vi "ELVIS III v1.0 Configure PWM.vi"(8 "error in (no error)":errorcluster, 9 "PWM Configuration":T4, 10 "PWM Channel":T1, 11 "myRIO Ref In":T2) -> (0 "error out":errorcluster, 2 "Max Counter Value":u16, 3 "Actual Frequency (Hz)":dbl)   [LabVIEW 2021]
uses:
  <vilib>/myRIO/Common/Instrument Driver Framework/myRIO v1.0/PWM/typedefs/PWM Configuration v1.0.ctl
  <vilib>/myRIO/Common/Instrument Driver Framework/Utilities/typedefs/myRIO v1.0 Reference.ctl
  <vilib>/myRIO/Common/Instrument Driver Framework/Utilities/typedefs/Generic FPGA Reference.ctl
  <vilib>/myRIO/Common/Instrument Driver Framework/myRIO v1.0/PWM/typedefs/PWM Channels Enum.ctl
  <vilib>/myRIO/Common/Instrument Driver Framework/ELVIS III v1.0/PWM/typedefs/ELVIS III PWM Channels FPGA Reference.ctl
  <vilib>/myRIO/Common/Instrument Driver Framework/Utilities/vis/Calculate Clock Settings.vi
  <vilib>/myRIO/Common/Instrument Driver Framework/Utilities/vis/Calculate TOP (Phase Correct Mode).vi
  <vilib>/myRIO/Common/Instrument Driver Framework/Utilities/vis/Calculate TOP (Normal Mode).vi
  <vilib>/myRIO/Common/Instrument Driver Framework/Utilities/vis/Calculate Frequency (Phase Correct Mode).vi
  <vilib>/myRIO/Common/Instrument Driver Framework/Utilities/vis/Calculate Frequency (Normal Mode).vi
  <vilib>/rvi/errors/niLvFpgaAdjustHostInterfaceError.vi
  <vilib>/rvi/interface/nirviReadWriteControl/nirviReadWriteControl.xnode
  NiFpgaLv.dll
  <vilib>/rvi/interface/Simulation/niFpgaSimulationCallBeginRW.vi
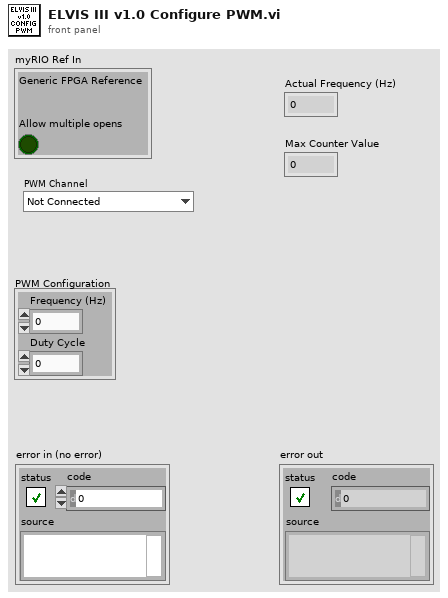
[diagram p1: front panel]
types:
  T1 = typedef "PWM Channels Enum.ctl" = enum16{"Not Connected", "C/PWM0", "C/PWM1", "A/PWM0", "A/PWM1", "A/PWM2", "A/PWM3", "A/PWM4", "A/PWM5", "A/PWM6", "A/PWM7", "A/PWM8", "A/PWM9", "A/PWM10", "A/PWM11", "A/PWM12", "A/PWM13", "A/PWM14", "A/PWM15", "A/PWM16", "A/PWM17", "A/PWM18", "A/PWM19", "B/PWM0", "B/PWM1", "B/PWM2", "B/PWM3", "B/PWM4", "B/PWM5", "B/PWM6", "B/PWM7", "B/PWM8", "B/PWM9", "B/PWM10", "B/PWM11", "B/PWM12", "B/PWM13", "B/PWM14", "B/PWM15", "B/PWM16", "B/PWM17", "B/PWM18", "B/PWM19", "PWM/PWM0", "PWM/PWM1", "PWM/PWM2", "PWM/PWM3", "PWM/PWM4", "PWM/PWM5", "PWM/PWM6", "PWM/PWM7", "PWM/PWM8", "PWM/PWM9"}
  T2 = typedef "myRIO v1.0 Reference.ctl" = cluster{"Generic FPGA Reference":T3, "Allow multiple opens":bool}
  T3 = typedef "Generic FPGA Reference.ctl" = refnum<k20>
  T4 = typedef "PWM Configuration v1.0.ctl" = cluster{"Frequency (Hz)":dbl, "Duty Cycle":dbl}
  T5 = typedef "ELVIS III PWM Channels FPGA Reference.ctl" = refnum<k20>
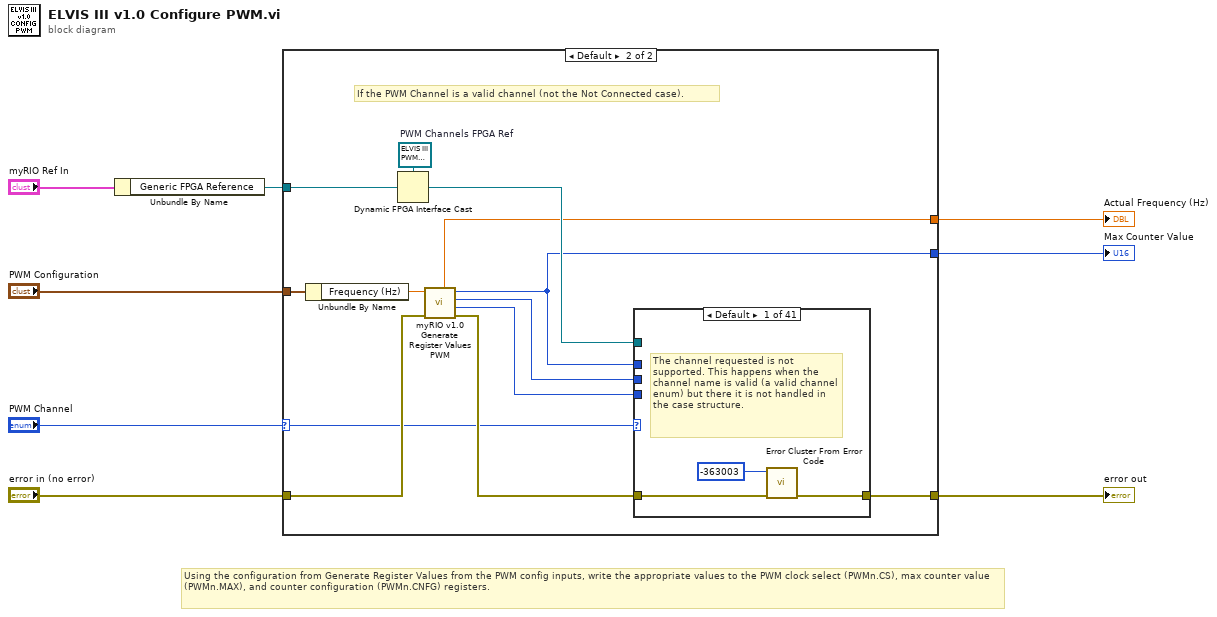
[diagram p0: block diagram]
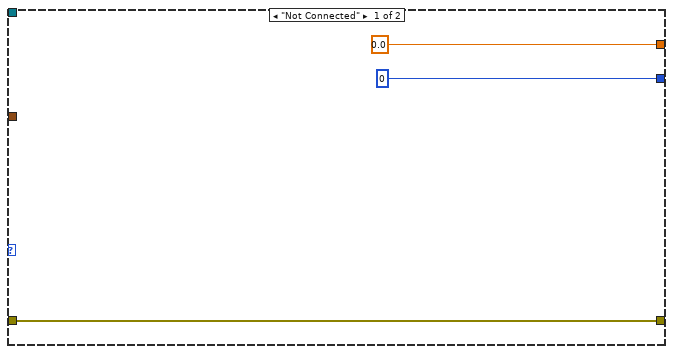
[diagram p2: hidden frame]
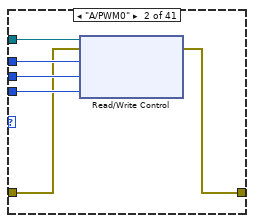
[diagram p3: hidden frame]
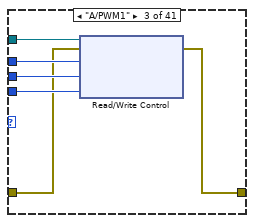
[diagram p4: hidden frame]
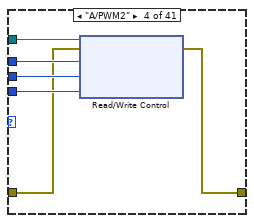
[diagram p5: hidden frame]
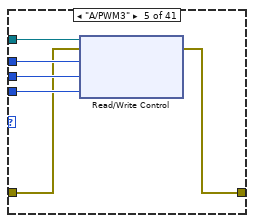
[diagram p6: hidden frame]
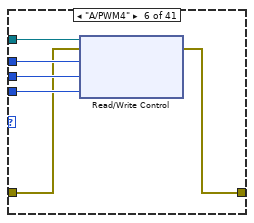
[diagram p7: hidden frame]
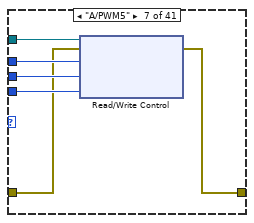
[diagram p8: hidden frame]
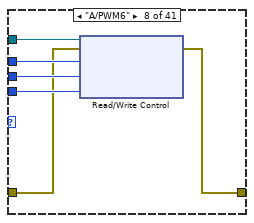
[diagram p9: hidden frame]
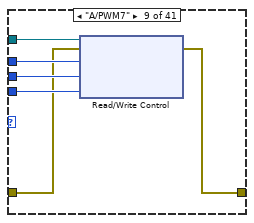
[diagram p10: hidden frame]
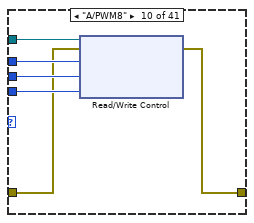
[diagram p11: hidden frame]
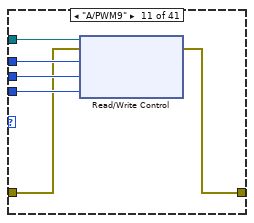
[diagram p12: hidden frame]
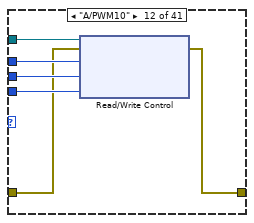
[diagram p13: hidden frame]
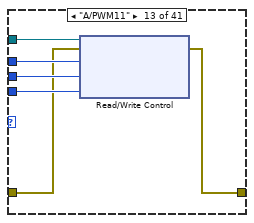
[diagram p14: hidden frame]
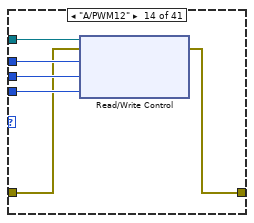
[diagram p15: hidden frame]
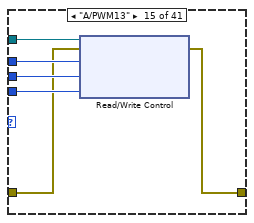
[diagram p16: hidden frame]
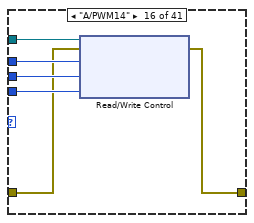
[diagram p17: hidden frame]
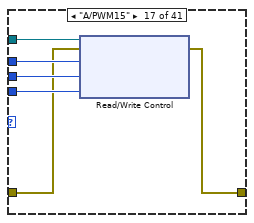
[diagram p18: hidden frame]
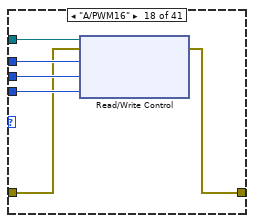
[diagram p19: hidden frame]
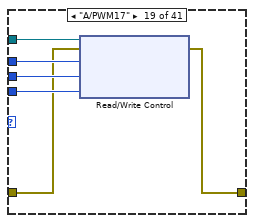
[diagram p20: hidden frame]
diagram:
  # "Using the configuration from Generate Register Values from the PWM config inputs, write the appropriate values to the PWM clock select (PWMn.CS), max counter value (PWMn.MAX), and counter configuration (PWMn.CNFG) registers."
  n1 = Unbundle By Name("myRIO Ref In") -> ("Generic FPGA Reference"=w1:T3)
  n2 = case shown="Default" "PWM Channel" {
    selector: "PWM Channel" -> [_ w12]
    tunnel: [w9 w22] -> w8
    tunnel: "PWM Configuration" -> [_ w14]
    tunnel: "error in (no error)" -> [w9 w16]
    tunnel: w1 -> [_ w21]
    tunnel: [u16 0 w19] -> w2
    tunnel: [0.0 ("Actual Frequency (Hz)") w20] -> w3
    frame "Not Connected" {
    }
    frame Default {
      w24 = T5 refnum  # PWM Channels FPGA Ref
      # "If the PWM Channel is a valid channel (not the Not Connected case)."
      n3 = Unbundle By Name(w14) -> ("Frequency (Hz)"=w13:dbl)
      n4 = Dynamic FPGA Interface Cast(Session In=w24, Type=w21) -> (Session Out=w23:T5)
      n5 = call <vilib>:"myRIO v1.0 Generate Register Values PWM.vi"("error in (no error)"=w16, "Frequency (Hz)"=w13) -> ("error out"=w15:errorcluster, "PWM.CS"=w17:u8, "PWM.CNFG"=w18:u8, "PWM.MAX"=w19:u16, "Actual Frequency (Hz)"=w20:dbl)  [unwired: 5 in]
      n6 = case shown="Default" w12 {
        tunnel: w23 -> [_ w33 w39 w45 w51 w57 w63 w69 w75 w81 w87 w93 w99 w105 w111 w117 w123 w129 w135 w141 w147 w153 w159 w165 w171 w177 w183 w189 w195 w201 w207 w213 w219 w225 w231 w237 w243 w249 w255 w261 w267]
        tunnel: [w25 w32 w38 w44 w50 w56 w62 w68 w74 w80 w86 w92 w98 w104 w110 w116 w122 w128 w134 w140 w146 w152 w158 w164 w170 w176 w182 w188 w194 w200 w206 w212 w218 w224 w230 w236 w242 w248 w254 w260 w266] -> w22
        tunnel: w19 -> [_ w31 w37 w43 w49 w55 w61 w67 w73 w79 w85 w91 w97 w103 w109 w115 w121 w127 w133 w139 w145 w151 w157 w163 w169 w175 w181 w187 w193 w199 w205 w211 w217 w223 w229 w235 w241 w247 w253 w259 w265]
        tunnel: w18 -> [_ w30 w36 w42 w48 w54 w60 w66 w72 w78 w84 w90 w96 w102 w108 w114 w120 w126 w132 w138 w144 w150 w156 w162 w168 w174 w180 w186 w192 w198 w204 w210 w216 w222 w228 w234 w240 w246 w252 w258 w264]
        tunnel: w17 -> [_ w29 w35 w41 w47 w53 w59 w65 w71 w77 w83 w89 w95 w101 w107 w113 w119 w125 w131 w137 w143 w149 w155 w161 w167 w173 w179 w185 w191 w197 w203 w209 w215 w221 w227 w233 w239 w245 w251 w257 w263]
        tunnel: w15 -> [w26 w28 w34 w40 w46 w52 w58 w64 w70 w76 w82 w88 w94 w100 w106 w112 w118 w124 w130 w136 w142 w148 w154 w160 w166 w172 w178 w184 w190 w196 w202 w208 w214 w220 w226 w232 w238 w244 w250 w256 w262]
        frame Default {
          # "The channel requested is not supported. This happens when the channel name is valid (a valid channel enum) but there it is not handled in the case structure."
          n7 = call <vilib>:"Error Cluster From Error Code.vi"("error in (no error)"=w26, "error code (0)"=-363003) -> ("error out"=w25:errorcluster)  [unwired: 7 in]
        }
        frame "A/PWM0" {
          n8 = xnode "Read/Write Control"("FPGA VI Reference In"=w33, "error in"=w28, "PWM.A_0.MAX"=w31, "PWM.A_0.CNFG"=w30, "PWM.A_0.CS"=w29) -> ("error out"=w32:errorcluster)  [unwired: 1 out]
        }
        frame "A/PWM1" {
          n9 = xnode "Read/Write Control"("FPGA VI Reference In"=w39, "error in"=w34, "PWM.A_1.MAX"=w37, "PWM.A_1.CNFG"=w36, "PWM.A_1.CS"=w35) -> ("error out"=w38:errorcluster)  [unwired: 1 out]
        }
        frame "A/PWM2" {
          n10 = xnode "Read/Write Control"("FPGA VI Reference In"=w45, "error in"=w40, "PWM.A_2.MAX"=w43, "PWM.A_2.CNFG"=w42, "PWM.A_2.CS"=w41) -> ("error out"=w44:errorcluster)  [unwired: 1 out]
        }
        frame "A/PWM3" {
          n11 = xnode "Read/Write Control"("FPGA VI Reference In"=w51, "error in"=w46, "PWM.A_3.MAX"=w49, "PWM.A_3.CNFG"=w48, "PWM.A_3.CS"=w47) -> ("error out"=w50:errorcluster)  [unwired: 1 out]
        }
        frame "A/PWM4" {
          n12 = xnode "Read/Write Control"("FPGA VI Reference In"=w57, "error in"=w52, "PWM.A_4.MAX"=w55, "PWM.A_4.CNFG"=w54, "PWM.A_4.CS"=w53) -> ("error out"=w56:errorcluster)  [unwired: 1 out]
        }
        frame "A/PWM5" {
          n13 = xnode "Read/Write Control"("FPGA VI Reference In"=w63, "error in"=w58, "PWM.A_5.MAX"=w61, "PWM.A_5.CNFG"=w60, "PWM.A_5.CS"=w59) -> ("error out"=w62:errorcluster)  [unwired: 1 out]
        }
        frame "A/PWM6" {
          n14 = xnode "Read/Write Control"("FPGA VI Reference In"=w69, "error in"=w64, "PWM.A_6.MAX"=w67, "PWM.A_6.CNFG"=w66, "PWM.A_6.CS"=w65) -> ("error out"=w68:errorcluster)  [unwired: 1 out]
        }
        frame "A/PWM7" {
          n15 = xnode "Read/Write Control"("FPGA VI Reference In"=w75, "error in"=w70, "PWM.A_7.MAX"=w73, "PWM.A_7.CNFG"=w72, "PWM.A_7.CS"=w71) -> ("error out"=w74:errorcluster)  [unwired: 1 out]
        }
        frame "A/PWM8" {
          n16 = xnode "Read/Write Control"("FPGA VI Reference In"=w81, "error in"=w76, "PWM.A_8.MAX"=w79, "PWM.A_8.CNFG"=w78, "PWM.A_8.CS"=w77) -> ("error out"=w80:errorcluster)  [unwired: 1 out]
        }
        frame "A/PWM9" {
          n17 = xnode "Read/Write Control"("FPGA VI Reference In"=w87, "error in"=w82, "PWM.A_9.MAX"=w85, "PWM.A_9.CNFG"=w84, "PWM.A_9.CS"=w83) -> ("error out"=w86:errorcluster)  [unwired: 1 out]
        }
        frame "A/PWM10" {
          n18 = xnode "Read/Write Control"("FPGA VI Reference In"=w93, "error in"=w88, "PWM.A_10.MAX"=w91, "PWM.A_10.CNFG"=w90, "PWM.A_10.CS"=w89) -> ("error out"=w92:errorcluster)  [unwired: 1 out]
        }
        frame "A/PWM11" {
          n19 = xnode "Read/Write Control"("FPGA VI Reference In"=w99, "error in"=w94, "PWM.A_11.MAX"=w97, "PWM.A_11.CNFG"=w96, "PWM.A_11.CS"=w95) -> ("error out"=w98:errorcluster)  [unwired: 1 out]
        }
        frame "A/PWM12" {
          n20 = xnode "Read/Write Control"("FPGA VI Reference In"=w105, "error in"=w100, "PWM.A_12.MAX"=w103, "PWM.A_12.CNFG"=w102, "PWM.A_12.CS"=w101) -> ("error out"=w104:errorcluster)  [unwired: 1 out]
        }
        frame "A/PWM13" {
          n21 = xnode "Read/Write Control"("FPGA VI Reference In"=w111, "error in"=w106, "PWM.A_13.MAX"=w109, "PWM.A_13.CNFG"=w108, "PWM.A_13.CS"=w107) -> ("error out"=w110:errorcluster)  [unwired: 1 out]
        }
        frame "A/PWM14" {
          n22 = xnode "Read/Write Control"("FPGA VI Reference In"=w117, "error in"=w112, "PWM.A_14.MAX"=w115, "PWM.A_14.CNFG"=w114, "PWM.A_14.CS"=w113) -> ("error out"=w116:errorcluster)  [unwired: 1 out]
        }
        frame "A/PWM15" {
          n23 = xnode "Read/Write Control"("FPGA VI Reference In"=w123, "error in"=w118, "PWM.A_15.MAX"=w121, "PWM.A_15.CNFG"=w120, "PWM.A_15.CS"=w119) -> ("error out"=w122:errorcluster)  [unwired: 1 out]
        }
        frame "A/PWM16" {
          n24 = xnode "Read/Write Control"("FPGA VI Reference In"=w129, "error in"=w124, "PWM.A_16.MAX"=w127, "PWM.A_16.CNFG"=w126, "PWM.A_16.CS"=w125) -> ("error out"=w128:errorcluster)  [unwired: 1 out]
        }
        frame "A/PWM17" {
          n25 = xnode "Read/Write Control"("FPGA VI Reference In"=w135, "error in"=w130, "PWM.A_17.MAX"=w133, "PWM.A_17.CNFG"=w132, "PWM.A_17.CS"=w131) -> ("error out"=w134:errorcluster)  [unwired: 1 out]
        }
        frame "A/PWM18" {
          n26 = xnode "Read/Write Control"("FPGA VI Reference In"=w141, "error in"=w136, "PWM.A_18.MAX"=w139, "PWM.A_18.CNFG"=w138, "PWM.A_18.CS"=w137) -> ("error out"=w140:errorcluster)  [unwired: 1 out]
        }
        frame "A/PWM19" {
          n27 = xnode "Read/Write Control"("FPGA VI Reference In"=w147, "error in"=w142, "PWM.A_19.MAX"=w145, "PWM.A_19.CNFG"=w144, "PWM.A_19.CS"=w143) -> ("error out"=w146:errorcluster)  [unwired: 1 out]
        }
        frame "B/PWM0" {
          n28 = xnode "Read/Write Control"("FPGA VI Reference In"=w153, "error in"=w148, "PWM.B_0.MAX"=w151, "PWM.B_0.CNFG"=w150, "PWM.B_0.CS"=w149) -> ("error out"=w152:errorcluster)  [unwired: 1 out]
        }
        frame "B/PWM1" {
          n29 = xnode "Read/Write Control"("FPGA VI Reference In"=w159, "error in"=w154, "PWM.B_1.MAX"=w157, "PWM.B_1.CNFG"=w156, "PWM.B_1.CS"=w155) -> ("error out"=w158:errorcluster)  [unwired: 1 out]
        }
        frame "B/PWM2" {
          n30 = xnode "Read/Write Control"("FPGA VI Reference In"=w165, "error in"=w160, "PWM.B_2.MAX"=w163, "PWM.B_2.CNFG"=w162, "PWM.B_2.CS"=w161) -> ("error out"=w164:errorcluster)  [unwired: 1 out]
        }
        frame "B/PWM3" {
          n31 = xnode "Read/Write Control"("FPGA VI Reference In"=w171, "error in"=w166, "PWM.B_3.MAX"=w169, "PWM.B_3.CNFG"=w168, "PWM.B_3.CS"=w167) -> ("error out"=w170:errorcluster)  [unwired: 1 out]
        }
        frame "B/PWM4" {
          n32 = xnode "Read/Write Control"("FPGA VI Reference In"=w177, "error in"=w172, "PWM.B_4.MAX"=w175, "PWM.B_4.CNFG"=w174, "PWM.B_4.CS"=w173) -> ("error out"=w176:errorcluster)  [unwired: 1 out]
        }
        frame "B/PWM5" {
          n33 = xnode "Read/Write Control"("FPGA VI Reference In"=w183, "error in"=w178, "PWM.B_5.MAX"=w181, "PWM.B_5.CNFG"=w180, "PWM.B_5.CS"=w179) -> ("error out"=w182:errorcluster)  [unwired: 1 out]
        }
        frame "B/PWM6" {
          n34 = xnode "Read/Write Control"("FPGA VI Reference In"=w189, "error in"=w184, "PWM.B_6.MAX"=w187, "PWM.B_6.CNFG"=w186, "PWM.B_6.CS"=w185) -> ("error out"=w188:errorcluster)  [unwired: 1 out]
        }
        frame "B/PWM7" {
          n35 = xnode "Read/Write Control"("FPGA VI Reference In"=w195, "error in"=w190, "PWM.B_7.MAX"=w193, "PWM.B_7.CNFG"=w192, "PWM.B_7.CS"=w191) -> ("error out"=w194:errorcluster)  [unwired: 1 out]
        }
        frame "B/PWM8" {
          n36 = xnode "Read/Write Control"("FPGA VI Reference In"=w201, "error in"=w196, "PWM.B_8.MAX"=w199, "PWM.B_8.CNFG"=w198, "PWM.B_8.CS"=w197) -> ("error out"=w200:errorcluster)  [unwired: 1 out]
        }
        frame "B/PWM9" {
          n37 = xnode "Read/Write Control"("FPGA VI Reference In"=w207, "error in"=w202, "PWM.B_9.MAX"=w205, "PWM.B_9.CNFG"=w204, "PWM.B_9.CS"=w203) -> ("error out"=w206:errorcluster)  [unwired: 1 out]
        }
        frame "B/PWM10" {
          n38 = xnode "Read/Write Control"("FPGA VI Reference In"=w213, "error in"=w208, "PWM.B_10.MAX"=w211, "PWM.B_10.CNFG"=w210, "PWM.B_10.CS"=w209) -> ("error out"=w212:errorcluster)  [unwired: 1 out]
        }
        frame "B/PWM11" {
          n39 = xnode "Read/Write Control"("FPGA VI Reference In"=w219, "error in"=w214, "PWM.B_11.MAX"=w217, "PWM.B_11.CNFG"=w216, "PWM.B_11.CS"=w215) -> ("error out"=w218:errorcluster)  [unwired: 1 out]
        }
        frame "B/PWM12" {
          n40 = xnode "Read/Write Control"("FPGA VI Reference In"=w225, "error in"=w220, "PWM.B_12.MAX"=w223, "PWM.B_12.CNFG"=w222, "PWM.B_12.CS"=w221) -> ("error out"=w224:errorcluster)  [unwired: 1 out]
        }
        frame "B/PWM13" {
          n41 = xnode "Read/Write Control"("FPGA VI Reference In"=w231, "error in"=w226, "PWM.B_13.MAX"=w229, "PWM.B_13.CNFG"=w228, "PWM.B_13.CS"=w227) -> ("error out"=w230:errorcluster)  [unwired: 1 out]
        }
        frame "B/PWM14" {
          n42 = xnode "Read/Write Control"("FPGA VI Reference In"=w237, "error in"=w232, "PWM.B_14.MAX"=w235, "PWM.B_14.CNFG"=w234, "PWM.B_14.CS"=w233) -> ("error out"=w236:errorcluster)  [unwired: 1 out]
        }
        frame "B/PWM15" {
          n43 = xnode "Read/Write Control"("FPGA VI Reference In"=w243, "error in"=w238, "PWM.B_15.MAX"=w241, "PWM.B_15.CNFG"=w240, "PWM.B_15.CS"=w239) -> ("error out"=w242:errorcluster)  [unwired: 1 out]
        }
        frame "B/PWM16" {
          n44 = xnode "Read/Write Control"("FPGA VI Reference In"=w249, "error in"=w244, "PWM.B_16.MAX"=w247, "PWM.B_16.CNFG"=w246, "PWM.B_16.CS"=w245) -> ("error out"=w248:errorcluster)  [unwired: 1 out]
        }
        frame "B/PWM17" {
          n45 = xnode "Read/Write Control"("FPGA VI Reference In"=w255, "error in"=w250, "PWM.B_17.MAX"=w253, "PWM.B_17.CNFG"=w252, "PWM.B_17.CS"=w251) -> ("error out"=w254:errorcluster)  [unwired: 1 out]
        }
        frame "B/PWM18" {
          n46 = xnode "Read/Write Control"("FPGA VI Reference In"=w261, "error in"=w256, "PWM.B_18.MAX"=w259, "PWM.B_18.CNFG"=w258, "PWM.B_18.CS"=w257) -> ("error out"=w260:errorcluster)  [unwired: 1 out]
        }
        frame "B/PWM19" {
          n47 = xnode "Read/Write Control"("FPGA VI Reference In"=w267, "error in"=w262, "PWM.B_19.MAX"=w265, "PWM.B_19.CNFG"=w264, "PWM.B_19.CS"=w263) -> ("error out"=w266:errorcluster)  [unwired: 1 out]
        }
      }
    }
  }
  "error out" <- w8
  "Actual Frequency (Hz)" <- w3
  "Max Counter Value" <- w2
